vi "CALC_FILT_GATE_TIME_TYPE.vi"(0 "VISA IN":refnum<visa-resource-name>, 1 "FilterType":string(combo), 5 "error in":errorcluster, 7 "Channel":i32) -> (14 "VISA Out":refnum<visa-resource-name>, 19 "error out":errorcluster)   [LabVIEW 2018, in "PNA-X.lvlib"]
doc: "CALCulate<cnum>:FILTer[:GATE]:TIME[:TYPE] <char> \n(Read-Write) Sets the type of gate filter used. \nSee Critical Note \nParameters \n<cnum> Channel number of the measurement. There must be a selected measurement \non that channel. If unspecified, <cnum> is set to 1. \n<char> Choose from: \nBPASs - Includes (passes) the range between the start and stop times. \nNOTCh - Excludes (attenuates) the range between the start and stop times. \nExamples CALC:FILT:TIME BPAS \ncalculate2:filter:gate:time:type notch \nQuery Syntax CALCulate<cnum>:FILTer[:GATE]:TIME[:TYPE]? \nReturn Type Character \nDefault BPAS \n1511\n\nCalculate:Format Command \nCritical Note: CALCulate commands act on the selected measurement. You can select one \nmeasurement for each channel using Calc:Par:Select \nSee Also \nExample using this command. \nLearn About Data Format \nSynchronizing the PNA and Controller"
uses:
  PNA-X.lvlib
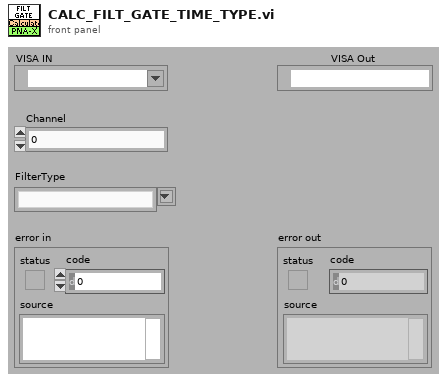
[diagram p1: front panel]
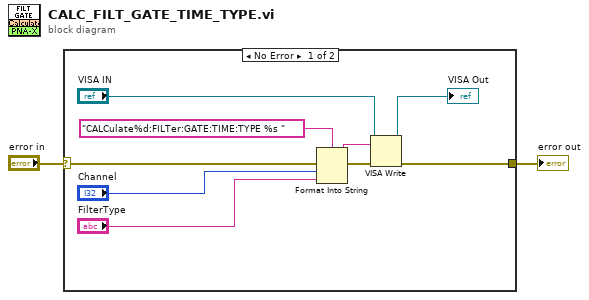
[diagram p0: block diagram]
diagram:
  n1 = case shown="No Error" "error in" {
    selector: "error in" -> [w11 w12]
    tunnel: [w6 w12] -> w1
    frame No Error {
      n2 = Format Into String(format string="CALCulate%d:FILTer:GATE:TIME:TYPE %s " ("Cmdline"), error in=w11, "Channel", "FilterType") -> (resulting string=w9:string, error out=w10:errorcluster)  [unwired: 1 in]
      n3 = VISA Write(VISA resource name="VISA IN", write buffer=w9, error in (no error)=w10) -> (VISA resource name out=→"VISA Out":refnum<visa-resource-name>, error out=w6:errorcluster)  [unwired: 1 out]
    }
    frame Error {
    }
  }
  "error out" <- w1
